vi "EAGLE GUI V6.vi"(9 "TableIn":string[][](table)) -> (1 "GUI Table":string[][](table), 2 "Exit":bool)   [LabVIEW 2015]
uses:
  Controls/Eagle Data.ctl
  Stream/Controls/RT Status Refs.ctl
  Stream/Robo Team Engine Command.ctl
  Stream/Robo Team Globals.vi
panel:
  in  "WB":bool
  out "error out":errorcluster
  out "Eagle Data":T1
  out "TableOut":string[][](table)
  out "ViewFinder Sign":picture
  out "Frame Rec":u32
  out "AlgoTime":u32
  out "FrameRate":dbl format="%#.1f"
  out "Stopped":bool
  in  "RangingNumeric":dbl
  in  "AimingNumeric":dbl
  in  "LEDRingNumeric":dbl
  in  "close":bool
  in  "Previous":bool
  in  "Next":bool
  in  "RangingSlider":dbl(slide)=1.0 caption="Ranging\nIntensity" max=10.0 step=1.0 scale=0.0..10.0
  in  "AimingSlider":dbl(slide)=1.0 caption="Aiming\nIntensity" max=10.0 step=1.0 scale=0.0..10.0
  in  "LEDRingSlider":dbl(slide)=1.0 caption="Illumination\nIntensity" max=10.0 step=1.0 scale=0.0..10.0
  out "Iris Found Status":bool
  in  "Tab":enum32{"Page 1", "Page 2", "Page 3"}(tab)
  out "Image":T2(plugin-control)
  # "Treatment Process"
  # "Treatment Info"
  # "Illumination Settings"
  # "Instructions"
  # "1. Adjust illumination\n2. Align the green cross to \n    the center of the pupil\n3. Form cross from the two\n    red lines (Ranging Beams)"
  # "Instructions"
  # "Limbus Border Found\nReady\nClick START"
  # "Instructions"
  # "READY!\n\nClick Start"
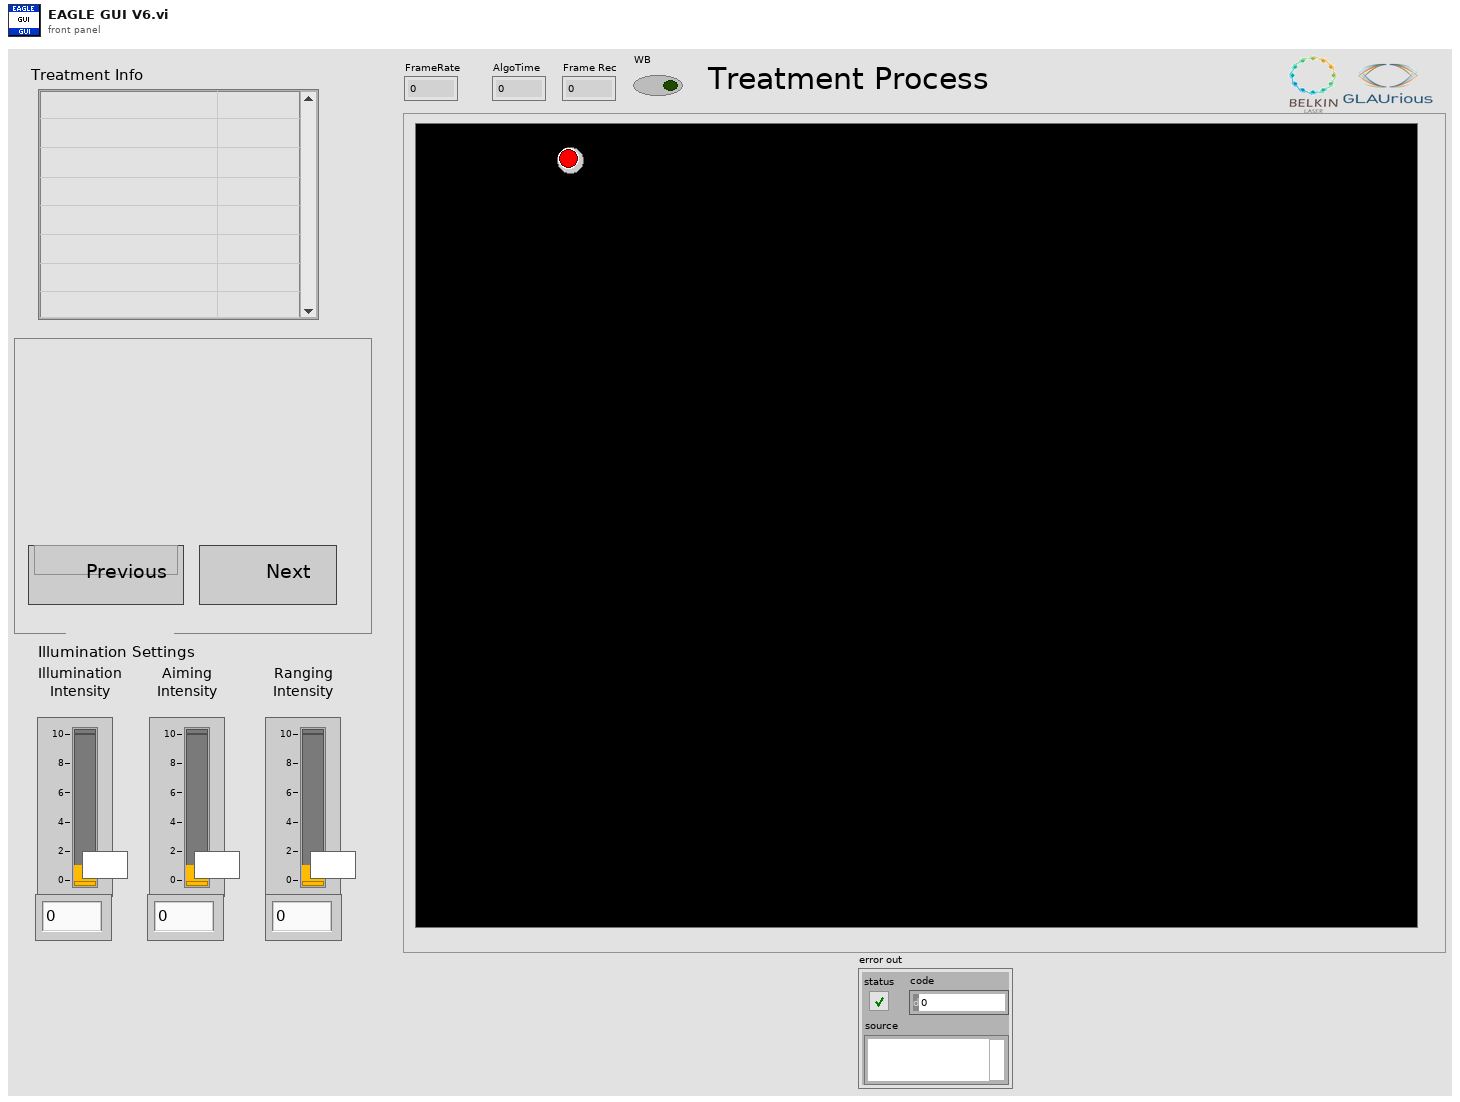
[diagram p1: front panel]
types:
  T1 = typedef "Eagle Data.ctl" = cluster{"Patient ID":string, "EyeSelect":enum32{"Right Eye", "Left Eye"}, "TreatArea":enum32{"Upper 180", "Lower 180", "Full 360"}, "EyeColor":enum32{"Dark", "Bright"}, "Laser Energy":dbl, "Number of pulses":u32, "Time between pulses":dbl, "Limbus distance":dbl, "Illumination Intensity":dbl, "Aiming Intensity":dbl, "Ranging Intensity":dbl}
  T2 = typedef "IMAQ Image.ctl" = refnum<image>
  T3 = typedef "RT Status Refs.ctl" = cluster{"Algo Time ref":refnum<vi>, "FrameRate ref":refnum<vi>, "FrameRecRef":refnum<vi>}
  T4 = typedef "Robo Team Engine Command.ctl" = cluster{"Command":string, "Data":variant, "Error":errorcluster, "Timeout":i32}
  T5 = enum8{"Enabled", "Disabled", "Disabled and Grayed Out"}
  T6 = typedef "LVPositionTypeDef.ctl" = cluster{"Left":i32, "Top":i32}
  T7 = typedef "LVRectTypeDef.ctl" = cluster{"Left":i16, "Top":i16, "Right":i16, "Bottom":i16}
  T8 = cluster{"Patient ID":string, "EyeSelect":enum32{"Right Eye", "Left Eye"}, "TreatArea":enum32{"Upper 180", "Lower 180", "Full 360"}, "EyeColor":enum32{"Dark", "Bright"}, "Laser Energy":dbl, "Number of pulses":u32, "Time between pulses":dbl, "Limbus distance":dbl, "LEDRingSlider":dbl, "AimingSlider":dbl, "RangingSlider":dbl}
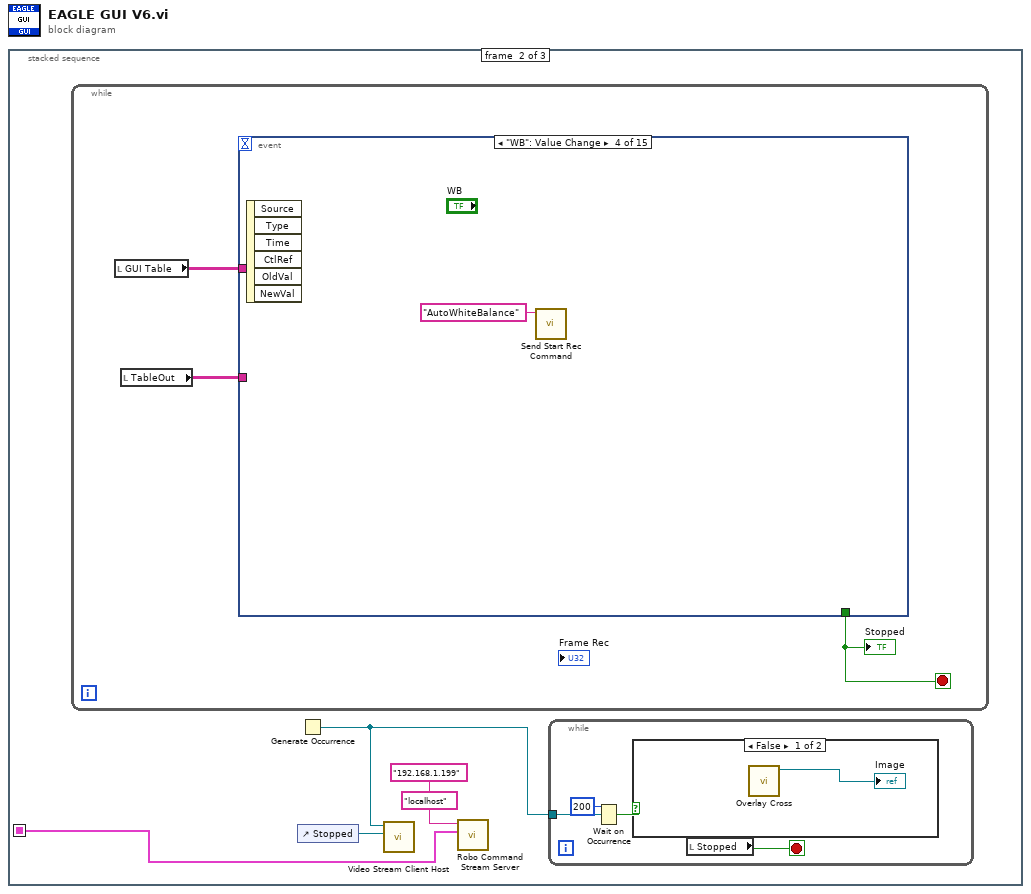
[diagram p0: block diagram]
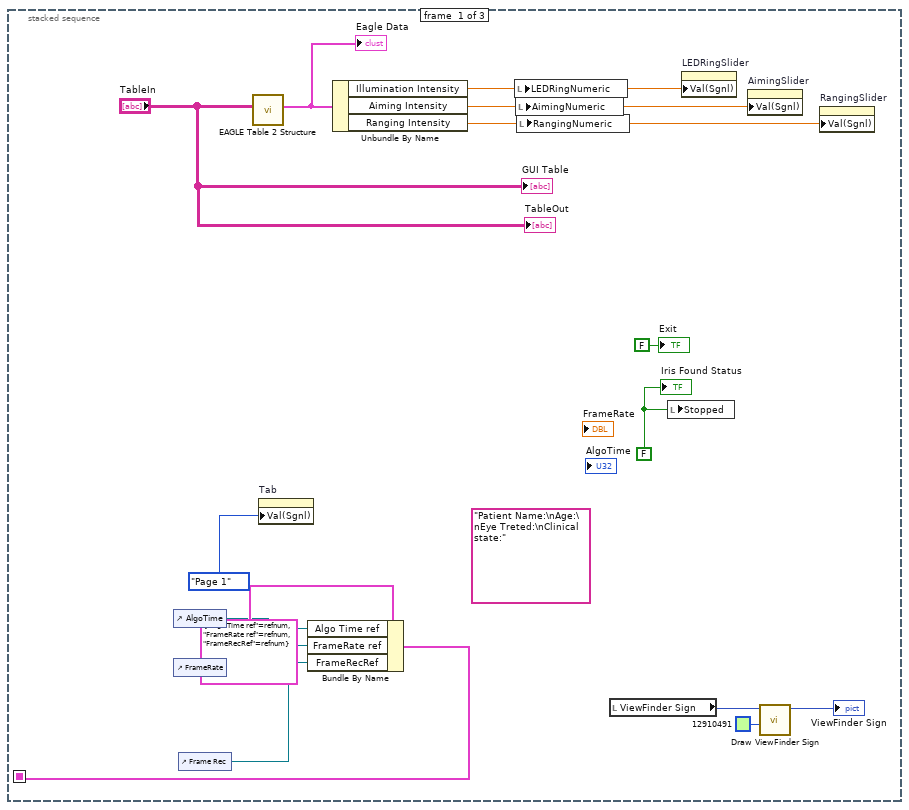
[diagram p2: hidden frame]
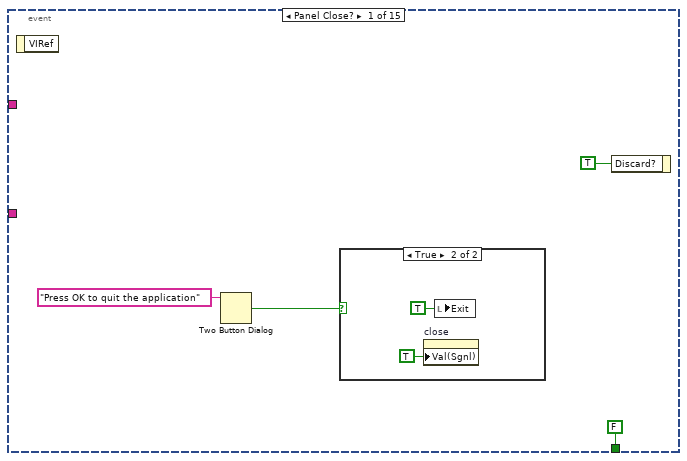
[diagram p4: hidden frame]
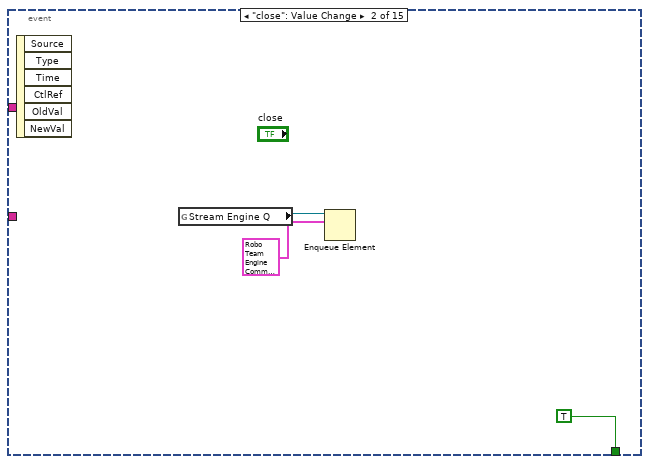
[diagram p6: hidden frame]
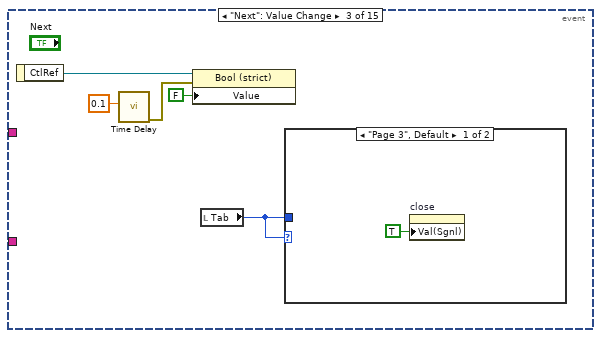
[diagram p7: hidden frame]
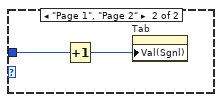
[diagram p8: hidden frame]
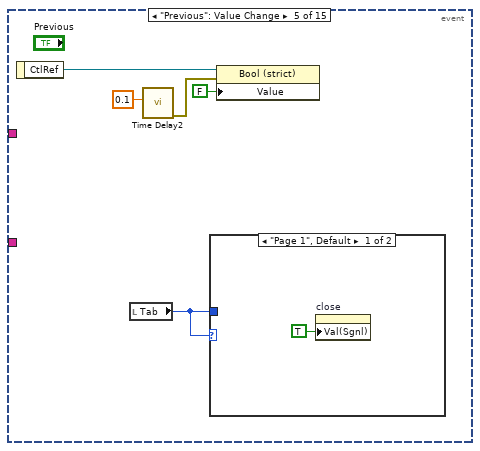
[diagram p9: hidden frame]
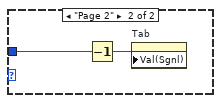
[diagram p10: hidden frame]
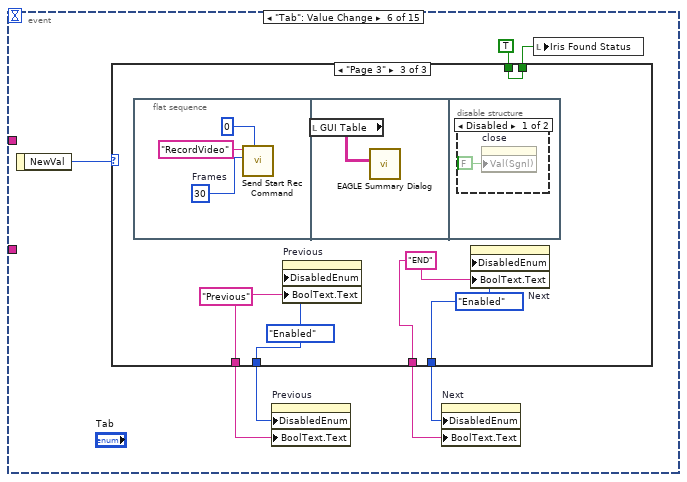
[diagram p11: hidden frame]
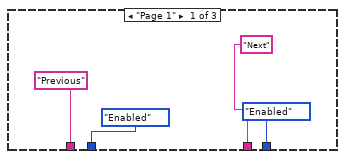
[diagram p12: hidden frame]
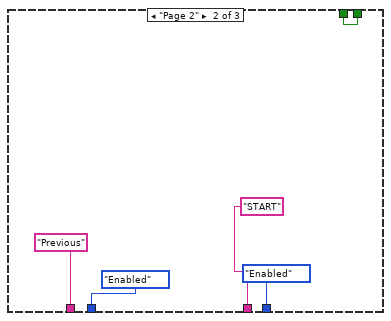
[diagram p13: hidden frame]
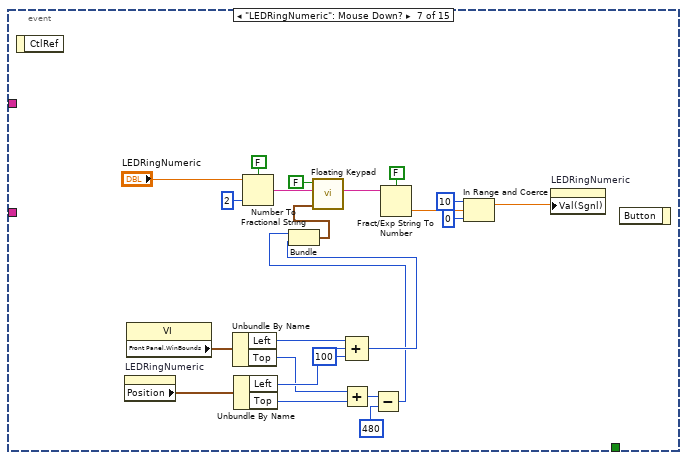
[diagram p15: hidden frame]
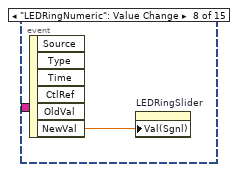
[diagram p16: hidden frame]
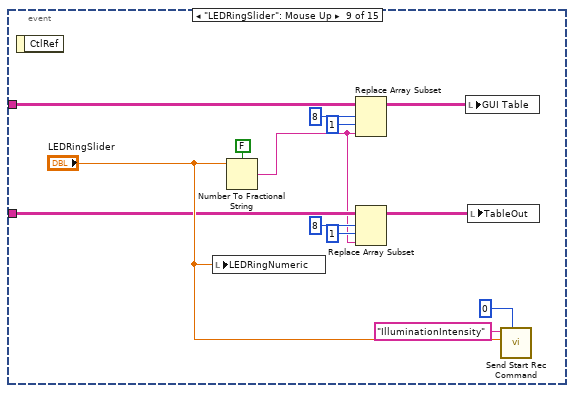
[diagram p17: hidden frame]
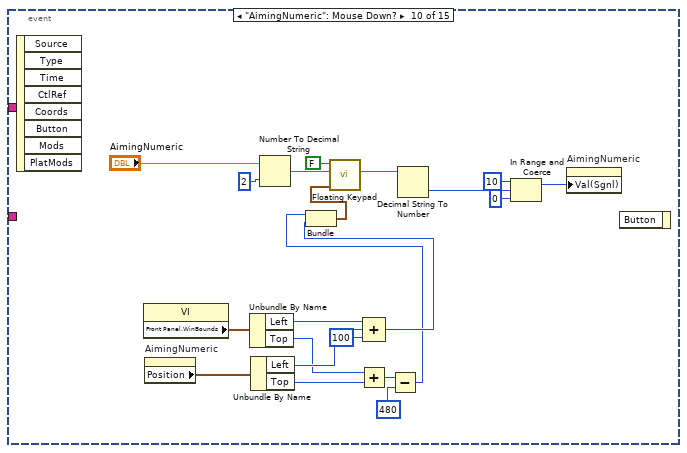
[diagram p18: hidden frame]
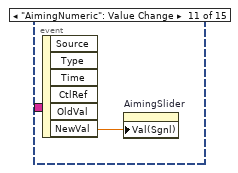
[diagram p19: hidden frame]
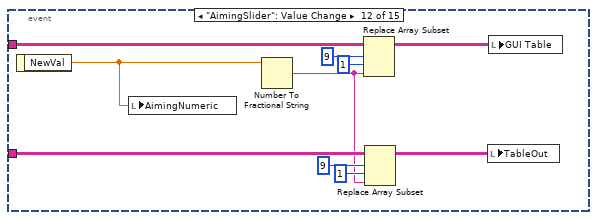
[diagram p20: hidden frame]
diagram:
  n1 = stacked-sequence {
    seq-local: [w13 _ _] -> [_ w18 _]
    frame #0 {
      w15 = FALSE ("Iris Found Status")
      (unwired) "Patient Name:\nAge:\nEye Treted:\nClinical state:" ("patient Info")
      n2 = control-ref of="AlgoTime"() -> (w11:refnum<vi>)
      n3 = control-ref of="FrameRate"() -> (w12:refnum<vi>)
      n4 = control-ref of="Frame Rec"() -> (w10:refnum<vi>)
      n5 = call "EAGLE Table 2 Structure.vi"("Table Control"="TableIn") -> ("Eagle Data"=w6:T1)  [unwired: 10 in]
      "Eagle Data" <- w6
      n6 = property on="Tab" class="TabCtl (strict)"("Val(Sgnl)"=enum32{"Page 1", "Page 2"}."Page 1" ("Tab")) -> ()  [unwired: 2 in, 2 out]
      n7 = Bundle By Name(cluster=T3 {"Algo Time ref"=refnum, "FrameRate ref"=refnum, "FrameRecRef"=refnum} ("StatusRefs"), "Algo Time ref"=w11, "FrameRate ref"=w12, "FrameRecRef"=w10) -> (w13:T3)
      n8 = Unbundle By Name(w6) -> ("Illumination Intensity"=w5:dbl, "Aiming Intensity"=w3:dbl, "Ranging Intensity"=w4:dbl)
      n9 = local write "LEDRingNumeric"(w5) -> ()
      n10 = local write "AimingNumeric"(w3) -> ()
      n11 = local write "RangingNumeric"(w4) -> ()
      n12 = local read "ViewFinder Sign"() -> (w9:picture)
      n13 = local write "Stopped"(w15) -> ()
      n14 = property on="LEDRingSlider" class="Slide (strict)"("Val(Sgnl)"=w5) -> ()  [unwired: 2 in, 2 out]
      n15 = property on="AimingSlider" class="Slide (strict)"("Val(Sgnl)"=w3) -> ()  [unwired: 2 in, 2 out]
      n16 = call "Draw ViewFinder Sign.vi"("Color"=u32 12910491, "2D Picture"=w9) -> ("2D Picture out"=→"ViewFinder Sign":picture)  [unwired: 9 in]
      n17 = property on="RangingSlider" class="Slide (strict)"("Val(Sgnl)"=w4) -> ()  [unwired: 2 in, 2 out]
      "Iris Found Status" <- w15
      "GUI Table" <- "TableIn"
      "TableOut" <- "TableIn"
      "Exit" <- FALSE ("Exit")
    }
    frame #1 {
      (unwired) "localhost" ("Controller IP")
      n18 = while {
        stop <- w28 stop-if-true
        n19 = local read "GUI Table"() -> (w27:string[][])
        n20 = local read "TableOut"() -> (w26:string[][])
        n21 = event shown="[3] \"WB\": Value Change" {
          selector: _ -> [_ _ _ _ _ _ _ _ _ _ _ _ _ _ _]
          dyn-events: _ -> [_ _ _ _ _ _ _ _ _ _ _ _ _ _ _]
          timeout: _ -> [_ _ _ _ _ _ _ _ _ _ _ _ _ _ _]
          tunnel: [FALSE TRUE _ _ _ _ _ _ _ _ _ _ _ _ _] -> w28
          tunnel: w27 -> [_ _ _ _ _ _ _ _ w111 _ _ w145 _ _ w180]
          tunnel: w26 -> [_ _ _ _ _ _ _ _ w107 _ _ w142 _ _ w177]
          event Panel Close? {
            n22 = event-data() -> ()  [unwired: 1 in, 1 out]
            n23 = Two Button Dialog(message="Press OK to quit the application") -> (T button?=w29:bool)  [unwired: 2 in]
            n24 = case shown="True" w29 {
              frame False {
              }
              frame True {
                n25 = property on="close" class="Bool (strict)"("Val(Sgnl)"=TRUE ("Value (Signaling)")) -> ()  [unwired: 2 in, 2 out]
                n26 = local write "Exit"(TRUE ("Exit")) -> ()
              }
            }
            n27 = event-data("Discard?"=TRUE) -> ()  [unwired: 1 in, 1 out]
          }
          event "close": Value Change {
            n28 = event-data() -> ()  [unwired: 1 in, 6 out]
            n29 = global read "Robo Team Globals.vi" "Stream Engine Q"() -> (w36:refnum<queue>)
            n30 = Enqueue Element(queue=w36, element=T4 {"Command"="Close", "Data"=variant, "Error"={"status"=FALSE, "code"=0, "source"=""}, "Timeout"=0}) -> ()  [unwired: 2 in, 3 out]
          }
          event "Next": Value Change {
            n31 = event-data() -> ("CtlRef"=w40:refnum<vi>)  [unwired: 1 in]
            n32 = call "Time Delay"("Delay Time (s)"=0.1) -> ("error out"=w39:errorcluster)  [unwired: 10 in]
            n33 = property class="Bool (strict)"(reference=w40, error in=w39, "Value"=FALSE) -> ()  [unwired: 2 out]
            n34 = local read "Tab"() -> (w42:enum32{"Page 1", "Page 2", "Page 3"})
            n35 = case shown="\"Page 3\", Default" w42 {
              tunnel: w42 -> [_ w44]
              frame "Page 3", Default {
                n36 = property on="close" class="Bool (strict)"("Val(Sgnl)"=TRUE ("Value (Signaling)")) -> ()  [unwired: 2 in, 2 out]
              }
              frame "Page 1", "Page 2" {
                n37 = Increment(x=w44) -> (x+1=w45:enum32{"Page 1", "Page 2", "Page 3"})
                n38 = property on="Tab" class="TabCtl (strict)"("Val(Sgnl)"=w45) -> ()  [unwired: 2 in, 2 out]
              }
            }
          }
          event "WB": Value Change {
            n39 = event-data() -> ()  [unwired: 1 in, 6 out]
            n40 = call "Send Start Rec Command.vi"("Command"="AutoWhiteBalance") -> ()  [unwired: 9 in, 2 out]
          }
          event "Previous": Value Change {
            n41 = event-data() -> ("CtlRef"=w47:refnum<vi>)  [unwired: 1 in]
            n42 = local read "Tab"() -> (w51:enum32{"Page 1", "Page 2", "Page 3"})
            n43 = call "Time Delay2"("Delay Time (s)"=0.1) -> ("error out"=w49:errorcluster)  [unwired: 10 in]
            n44 = case shown="\"Page 1\", Default" w51 {
              tunnel: w51 -> [_ w54]
              frame "Page 1", Default {
                n45 = property on="close" class="Bool (strict)"("Val(Sgnl)"=TRUE ("Value (Signaling)")) -> ()  [unwired: 2 in, 2 out]
              }
              frame "Page 2" {
                n46 = Decrement(x=w54) -> (x-1=w53:enum32{"Page 1", "Page 2", "Page 3"})
                n47 = property on="Tab" class="TabCtl (strict)"("Val(Sgnl)"=w53) -> ()  [unwired: 2 in, 2 out]
              }
            }
            n48 = property class="Bool (strict)"(reference=w47, error in=w49, "Value"=FALSE) -> ()  [unwired: 2 out]
          }
          event "Tab": Value Change {
            n49 = event-data() -> ("NewVal"=w61:enum32{"Page 1", "Page 2", "Page 3"})  [unwired: 1 in]
            n50 = case shown="\"Page 3\"" w61 {
              tunnel: [T5."Enabled" ("Disabled") T5."Enabled" ("Disabled") w71] -> w60
              tunnel: [T5."Enabled" ("Disabled") T5."Enabled" ("Disabled") w73] -> w59
              tunnel: ["Next" "START" w74] -> w58
              tunnel: ["Previous" "Previous" w72] -> w57
              tunnel: [_ w66 w75] -> w56
              tunnel: TRUE -> [_ w66 w75]
              frame "Page 1" {
              }
              frame "Page 2" {
              }
              frame "Page 3" {
                w72 = "Previous"
                w74 = "END"
                w71 = T5."Enabled" ("Disabled")
                w73 = T5."Enabled" ("Disabled")
                n51 = flat-sequence {
                  frame #0 {
                    w77 = 30  # Frames
                    n52 = call "Send Start Rec Command.vi"("timeout in ms (5000)"=0, "Data in"=w77, "Command"="RecordVideo") -> ()  [unwired: 7 in, 2 out]
                  }
                  frame #1 {
                    n53 = local read "GUI Table"() -> (w79:string[][])
                    n54 = call "EAGLE Summary Dialog.vi"("Table Control in"=w79) -> ()  [unwired: 11 in]
                  }
                  frame #2 {
                    n55 = disable-structure shown="Disabled" {
                      frame Disabled {
                        n56 = property on="close" class="Bool (strict)"("Val(Sgnl)"=FALSE ("Value (Signaling)")) -> ()  [unwired: 2 in, 2 out]
                      }
                      frame Enabled {
                      }
                    }
                  }
                }
                n57 = property on="Previous" class="Bool (strict)"("DisabledEnum"=w71, "BoolText.Text"=w72) -> ()  [unwired: 2 in, 2 out]
                n58 = property on="Next" class="Bool (strict)"("DisabledEnum"=w73, "BoolText.Text"=w74) -> ()  [unwired: 2 in, 2 out]
              }
            }
            n59 = property on="Previous" class="Bool (strict)"("DisabledEnum"=w60, "BoolText.Text"=w57) -> ()  [unwired: 2 in, 2 out]
            n60 = property on="Next" class="Bool (strict)"("DisabledEnum"=w59, "BoolText.Text"=w58) -> ()  [unwired: 2 in, 2 out]
            n61 = local write "Iris Found Status"(w56) -> ()
          }
          event "LEDRingNumeric": Mouse Down? {
            n62 = event-data() -> ()  [unwired: 1 in, 1 out]
            n63 = property on="LEDRingNumeric" class="DigNum (strict)"() -> ("Position"=w88:T6)  [unwired: 2 in, 2 out]
            n64 = property class="VI"() -> ("Front Panel.WinBounds"=w87:T7)  [unwired: 2 in, 2 out]
            n65 = Unbundle By Name(w87) -> ("Left"=w100:i16, "Top"=w97:i16)
            n66 = Unbundle By Name(w88) -> ("Left"=w99:i32, "Top"=w98:i32)
            n67 = Number To Fractional String(use system decimal point (T)=FALSE, number="LEDRingNumeric", precision (6)=i16 2) -> (F-format string=w103:string)  [unwired: 1 in]
            n68 = Add(x=w97, y=w98) -> (x+y=w94:i32)
            n69 = Compound Arithmetic op=ADD(w100, w99, 100 ("value")) -> (w95:i32)
            n70 = Subtract(x=w94, y=480) -> (x-y=w92:i32)
            n71 = Bundle(w92, w95) -> (w91:cluster{i32, i32})  [unwired: 1 in]
            n72 = call "Floating Keypad.vi"("Position"=w91, "StringIn"=w103, "Allow dot"=FALSE) -> ("StringOut"=w102:string)  [unwired: 8 in]
            n73 = Fract/Exp String To Number(use system decimal point (T)=FALSE, string=w102) -> (number=w86:dbl)  [unwired: 2 in, 1 out]
            n74 = In Range and Coerce(upper limit=10, x=w86, lower limit=0) -> (coerced(x)=w85:dbl)  [unwired: 1 out]
            n75 = property on="LEDRingNumeric" class="DigNum (strict)"("Val(Sgnl)"=w85) -> ()  [unwired: 2 in, 2 out]
            n76 = event-data() -> ()  [unwired: 2 in, 1 out]
          }
          event "LEDRingNumeric": Value Change {
            n77 = event-data() -> ("NewVal"=w104:dbl)  [unwired: 1 in, 5 out]
            n78 = property on="LEDRingSlider" class="Slide (strict)"("Val(Sgnl)"=w104) -> ()  [unwired: 2 in, 2 out]
          }
          event "LEDRingSlider": Mouse Up {
            n79 = event-data() -> ()  [unwired: 1 in, 1 out]
            n80 = local write "LEDRingNumeric"("LEDRingSlider") -> ()
            n81 = Number To Fractional String(use system decimal point (T)=FALSE, number="LEDRingSlider") -> (F-format string=w106:string)  [unwired: 2 in]
            n82 = Replace Array Subset(array=w111, new element=w106, index (row)=8 ("disabled index (row)"), index (col)=1 ("disabled index (col)")) -> (w117:string[][])
            n83 = Replace Array Subset(array=w107, new element=w106, index (row)=8 ("disabled index (row)"), index (col)=1 ("disabled index (col)")) -> (w105:string[][])
            n84 = local write "GUI Table"(w117) -> ()
            n85 = local write "TableOut"(w105) -> ()
            n86 = call "Send Start Rec Command.vi"("timeout in ms (5000)"=0, "Data in"="LEDRingSlider", "Command"="IlluminationIntensity") -> ()  [unwired: 7 in, 2 out]
          }
          event "AimingNumeric": Mouse Down? {
            n87 = event-data() -> ()  [unwired: 1 in, 8 out]
            n88 = property class="VI"() -> ("Front Panel.WinBounds"=w122:T7)  [unwired: 2 in, 2 out]
            n89 = property on="AimingNumeric" class="DigNum (strict)"() -> ("Position"=w123:T6)  [unwired: 2 in, 2 out]
            n90 = Unbundle By Name(w122) -> ("Left"=w135:i16, "Top"=w132:i16)
            n91 = Unbundle By Name(w123) -> ("Left"=w134:i32, "Top"=w133:i32)
            n92 = Number To Decimal String(number="AimingNumeric", width (-)=i16 2 ("precision (6)")) -> (decimal integer string=w138:string)
            n93 = Add(x=w132, y=w133) -> (x+y=w129:i32)
            n94 = Compound Arithmetic op=ADD(w135, w134, 100 ("value")) -> (w130:i32)
            n95 = Subtract(x=w129, y=480) -> (x-y=w127:i32)
            n96 = Bundle(w127, w130) -> (w126:cluster{i32, i32})  [unwired: 1 in]
            n97 = call "Floating Keypad.vi"("Position"=w126, "StringIn"=w138, "Allow dot"=FALSE) -> ("StringOut"=w137:string)  [unwired: 8 in]
            n98 = Decimal String To Number(string=w137) -> (number=w119:i32)  [unwired: 2 in, 1 out]
            n99 = In Range and Coerce(upper limit=10, x=w119, lower limit=0) -> (coerced(x)=w118:i32)  [unwired: 1 out]
            n100 = property on="AimingNumeric" class="DigNum (strict)"("Val(Sgnl)"=w118) -> ()  [unwired: 2 in, 2 out]
            n101 = event-data() -> ()  [unwired: 2 in, 1 out]
          }
          event "AimingNumeric": Value Change {
            n102 = event-data() -> ("NewVal"=w139:dbl)  [unwired: 1 in, 5 out]
            n103 = property on="AimingSlider" class="Slide (strict)"("Val(Sgnl)"=w139) -> ()  [unwired: 2 in, 2 out]
          }
          event "AimingSlider": Value Change {
            n104 = event-data() -> ("NewVal"=w146:dbl)  [unwired: 1 in]
            n105 = local write "AimingNumeric"(w146) -> ()
            n106 = Number To Fractional String(number=w146) -> (F-format string=w141:string)  [unwired: 3 in]
            n107 = Replace Array Subset(array=w145, new element=w141, index (row)=9 ("disabled index (row)"), index (col)=1 ("disabled index (col)")) -> (w149:string[][])
            n108 = Replace Array Subset(array=w142, new element=w141, index (row)=9 ("disabled index (row)"), index (col)=1 ("disabled index (col)")) -> (w140:string[][])
            n109 = local write "TableOut"(w140) -> ()
            n110 = local write "GUI Table"(w149) -> ()
          }
          event "RangingNumeric": Mouse Down? {
            n111 = event-data() -> ()  [unwired: 1 in, 8 out]
            n112 = property class="VI"() -> ("Front Panel.WinBounds"=w156:T7)  [unwired: 2 in, 2 out]
            n113 = property on="RangingNumeric" class="DigNum (strict)"() -> ("Position"=w157:T6)  [unwired: 2 in, 2 out]
            n114 = Unbundle By Name(w156) -> ("Left"=w169:i16, "Top"=w166:i16)
            n115 = Unbundle By Name(w157) -> ("Left"=w168:i32, "Top"=w167:i32)
            n116 = Number To Fractional String(use system decimal point (T)=FALSE, number="RangingNumeric", precision (6)=i16 2) -> (F-format string=w172:string)  [unwired: 1 in]
            n117 = Add(x=w166, y=w167) -> (x+y=w163:i32)
            n118 = Compound Arithmetic op=ADD(w169, w168, 100 ("value")) -> (w164:i32)
            n119 = Subtract(x=w163, y=480) -> (x-y=w161:i32)
            n120 = Bundle(w161, w164) -> (w160:cluster{i32, i32})  [unwired: 1 in]
            n121 = call "Floating Keypad.vi"("Position"=w160, "StringIn"=w172, "Allow dot"=FALSE) -> ("StringOut"=w171:string)  [unwired: 8 in]
            n122 = Fract/Exp String To Number(use system decimal point (T)=FALSE, string=w171) -> (number=w153:dbl)  [unwired: 2 in, 1 out]
            n123 = In Range and Coerce(upper limit=10, x=w153, lower limit=0) -> (coerced(x)=w152:dbl)  [unwired: 1 out]
            n124 = property on="RangingNumeric" class="DigNum (strict)"("Val(Sgnl)"=w152) -> ()  [unwired: 2 in, 2 out]
            n125 = event-data() -> ()  [unwired: 2 in, 1 out]
          }
          event "RangingNumeric": Value Change {
            n126 = event-data() -> ("NewVal"=w173:dbl)  [unwired: 1 in, 5 out]
            n127 = property on="RangingSlider" class="Slide (strict)"("Val(Sgnl)"=w173) -> ()  [unwired: 2 in, 2 out]
          }
          event "RangingSlider": Value Change {
            n128 = event-data() -> ("NewVal"=w181:dbl)  [unwired: 1 in]
            n129 = local write "RangingNumeric"(w181) -> ()
            n130 = Number To Decimal String(number=w181) -> (decimal integer string=w175:string)  [unwired: 1 in]
            n131 = Replace Array Subset(array=w180, new element=w175, index (row)=10 ("disabled index (row)"), index (col)=1 ("disabled index (col)")) -> (w183:string[][])
            n132 = Replace Array Subset(array=w177, new element=w175, index (row)=10 ("disabled index (row)"), index (col)=1 ("disabled index (col)")) -> (w174:string[][])
            n133 = local write "GUI Table"(w183) -> ()
            n134 = local write "TableOut"(w174) -> ()
          }
        }
        "Stopped" <- w28
      }
      n135 = Generate Occurrence() -> (w19:refnum<k4>)
      n136 = control-ref of="Stopped"() -> (w20:refnum<vi>)
      n137 = call "Video Stream Client Host.vi"("Close ref"=w20, "occurrence"=w19) -> ()  [unwired: 10 in]
      n138 = call "Robo Command Stream Server.vi"("StatusRefs"=w18, "Controller IP"="192.168.1.199") -> ()  [unwired: 10 in]
      n139 = while {
        tunnel: w19 -> [w23]
        stop <- w24 stop-if-true
        n140 = Wait on Occurrence(2:w23, 3:200 ("ms timeout (-1)")) -> (0:w21:bool)  [unwired: 1 in]
        n141 = case shown="False" w21 {
          frame False {
            n142 = call "Overlay Cross.vi"() -> ("Image Out"=→"Image":T2)  [unwired: 11 in]
          }
          frame True {
          }
        }
        n143 = local read "Stopped"() -> (w24:bool)
      }
    }
    frame #2 {
      n144 = local read "Eagle Data"() -> (w204:T1)
      n145 = Unbundle By Name(w204) -> ("Patient ID"=w203:string, "EyeSelect"=w202:enum32{"Right Eye", "Left Eye"}, "TreatArea"=w201:enum32{"Upper 180", "Lower 180", "Full 360"}, "EyeColor"=w200:enum32{"Dark", "Bright"}, "Laser Energy"=w199:dbl, "Number of pulses"=w198:u32, "Time between pulses"=w197:dbl, "Limbus distance"=w196:dbl)
      n146 = local read "LEDRingSlider"() -> (w195:dbl)
      n147 = call <vilib>:"Application Directory.vi"() -> ("Application Directory"=w191:path)
      n148 = Build Path(base path=w191, name or relative path="EAGLE GUI Data.dat") -> (appended path=w185:path)
      n149 = Bundle("Patient ID"=w203, "EyeSelect"=w202, "TreatArea"=w201, "EyeColor"=w200, "Laser Energy"=w199, "Number of pulses"=w198, "Time between pulses"=w197, "Limbus distance"=w196, "LEDRingSlider"=w195, "AimingSlider"="AimingSlider", "RangingSlider"="RangingSlider") -> (w192:T8)  [unwired: 1 in]
      n150 = call "EAGLE Structure 2 Table.vi"("Eagle Data"=w192) -> ("TableOut"=w189:string[][])  [unwired: 10 in]
      n151 = Array To Spreadsheet String(delimiter (Tab)=",", array=w189, 3:"%s" ("format string")) -> (spreadsheet string=w186:string)
      n152 = Write to Text File(file (use dialog)=w185, text=w186) -> (error out=→"error out":errorcluster)  [unwired: 2 in, 2 out]
    }
  }
